vi "FestoCPX.File.Write.vi"(8 "error in":errorcluster, 11 "Settings dir":path) -> (0 "error out":errorcluster)   [LabVIEW 2016]
uses:
  FestoCPX.DO.Signal.ctl
  FestoCPX.DI.Signal.ctl
  FestoCPX.Global.vi
  <vilib>/Utility/config.llb/Write Key (I32).vi
  <vilib>/Utility/config.llb/Write Key (String).vi
  <vilib>/Utility/config.llb/NI_LVConfig.lvlib
panel:
  in  "DI Signal":T1
  in  "DO Signal":T2
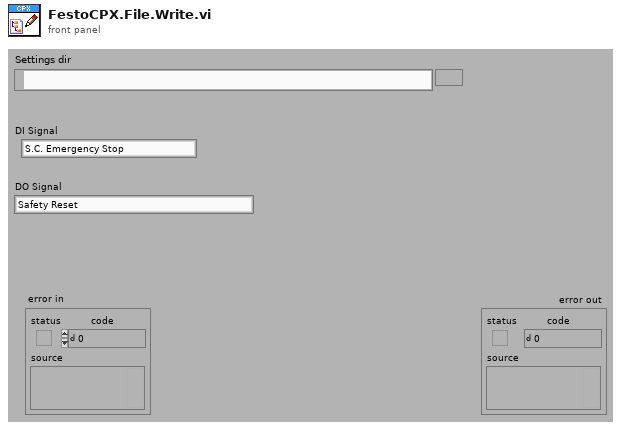
[diagram p1: front panel]
types:
  T1 = typedef "FestoCPX.DI.Signal.ctl" = enum16{"S.C. Emergency Stop", "S.C. Side Door Close", "S.C. Front Door Close", "S.C. Front Door Secured", "Button Start", "Button Stop", "Button Control", "Product Move Home", "Product Move Work", "Table Position", "Table Lock", "Product Lift A Home", "Product Lift B Home", "Product Arm OK", "Product Arm NOK", "Product Arm Work", "Revolver ID 1", "Revolver ID 2", "Revolver ID 3", "Revolver ID 4", "Revolver ID 5", "Air Pressure Inside", "Air Pressure Inlet", "Product Slot 1 A Present", "Product Slot 1 B Present", "Product Slot 2 A Present", "Product Slot 2 B Present", "Product Slot 3 A Present", "Product Slot 3 B Present", "Product Slot 4 A Present", "Product Slot 4 B Present", "Product Final A Present", "Product Final B Present", "Product Output A Present", "Product Output B Present", "Product Container OK Present", "Product Container NOK Present", "Fork ID 1", "Fork ID 2"}
  T2 = typedef "FestoCPX.DO.Signal.ctl" = enum16{"Safety Reset", "Air Main Valve", "Door Lock", "Button LED Start", "Button LED Stop", "Button LED Control", "Traffic LED Red", "Traffic LED Orange", "Traffic LED Green", "Horn", "Laser Interlock", "Laser Trigger", "Laser Fume Extractor", "Product Suction Gripper Slot 1 A", "Product Suction Gripper Slot 1 B", "Product Suction Gripper Slot 2 A", "Product Suction Gripper Slot 2 B", "Product Suction Gripper Slot 3 A", "Product Suction Gripper Slot 3 B", "Product Suction Gripper Slot 4 A", "Product Suction Gripper Slot 4 B", "Product Suction Gripper Final A", "Product Suction Gripper Final B", "Lamp", "Q1 Product Move Work", "Q1 Product Move Home", "Q2 Table Turn Work", "Q2 Table Turn Home", "Q3 Product Lift A", "Q3 Product Lift B", "Q4 Product Arm OK", "Q4 Product Arm NOK", "Q5 Product Arm Work", "Q6 Product BlowOut A", "Q6 Product BlowOut B"}
  T3 = typedef "FestoCPX.Data.Sets.ctl" = cluster{"IP":string, "Timeout_ms":i32, "ReconnectPeriod_s":i32, "Config.DI":T4[], "Config.DO":T6[]}
  T4 = typedef "FestoCPX.DI.Sets.ctl" = cluster{"Name":string, "Channel":T5, "Negate":bool}
  T5 = typedef "FestoCPX.DI.ctl" = enum16{"0.0", "0.1", "0.2", "0.3", "0.4", "0.5", "0.6", "0.7", "1.0", "1.1", "1.2", "1.3", "1.4", "1.5", "1.6", "1.7", "2.0", "2.1", "2.2", "2.3", "2.4", "2.5", "2.6", "2.7", "3.0", "3.1", "3.2", "3.3", "3.4", "3.5", "3.6", "3.7", "4.0", "4.1", "4.2", "4.3", "4.4", "4.5", "4.6", "4.7"}
  T6 = typedef "FestoCPX.DO.Sets.ctl" = cluster{"Name":string, "Channel":T7, "Negate":bool, "Default":bool}
  T7 = typedef "FestoCPX.DO.ctl" = enum16{"4.0", "4.1", "4.2", "4.3", "4.4", "4.5", "4.6", "4.7", "5.0", "5.1", "5.2", "5.3", "5.4", "5.5", "5.6", "5.7", "6.0", "6.1", "6.2", "6.3", "6.4", "6.5", "6.6", "6.7", "Q1K1", "Q1K2", "Q2K1", "Q2K2", "Q3K1", "Q3K2", "Q4K1", "Q4K2", "Q5K1", "Q5K2", "Q6K1", "Q6K2"}
  T8 = typedef "NI_LVConfig.lvlib/Config Data RefNum.ctl" = refnum<k1>
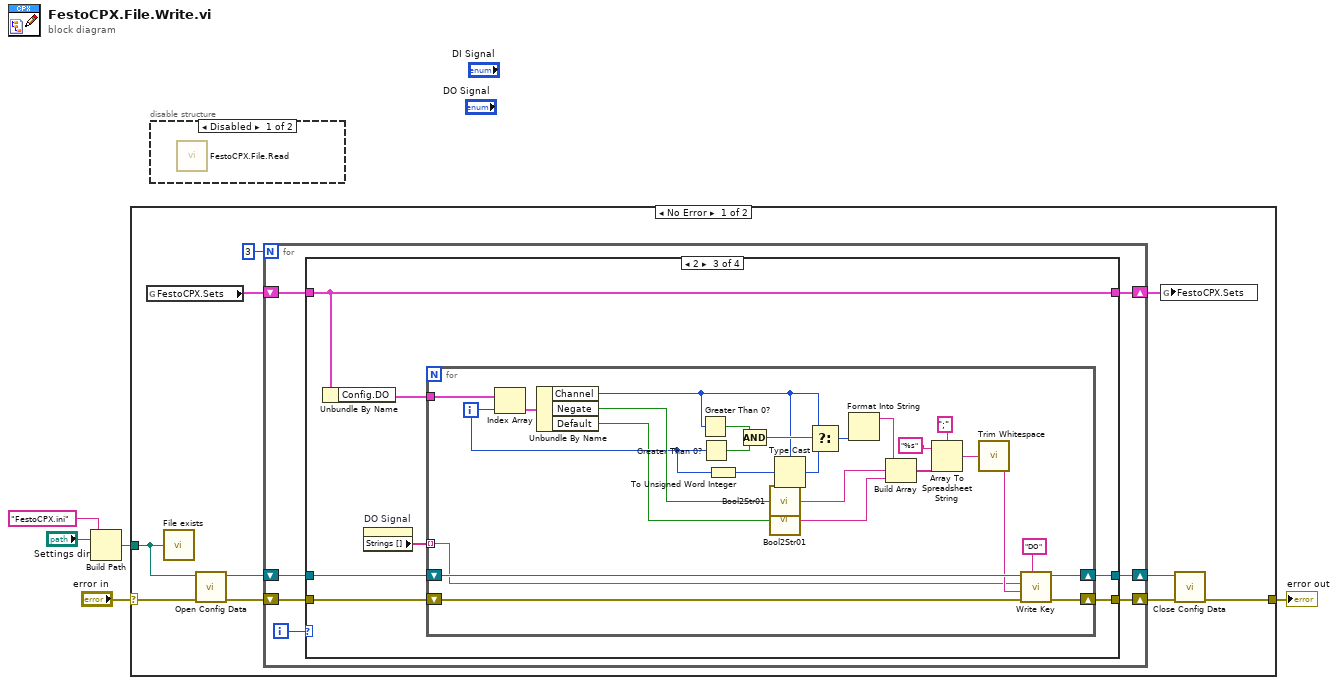
[diagram p0: block diagram]
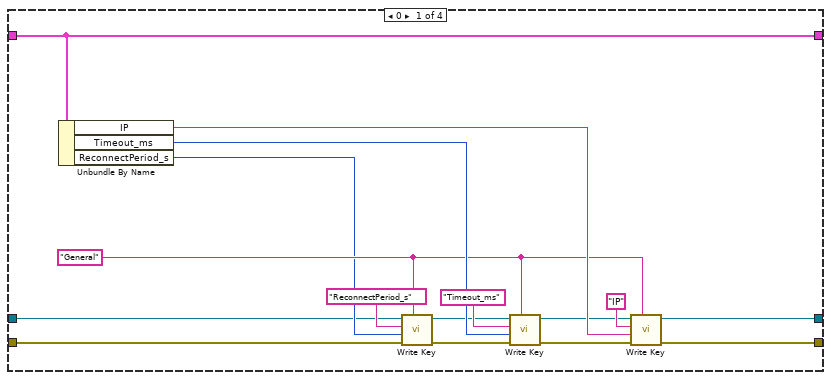
[diagram p3: hidden frame]
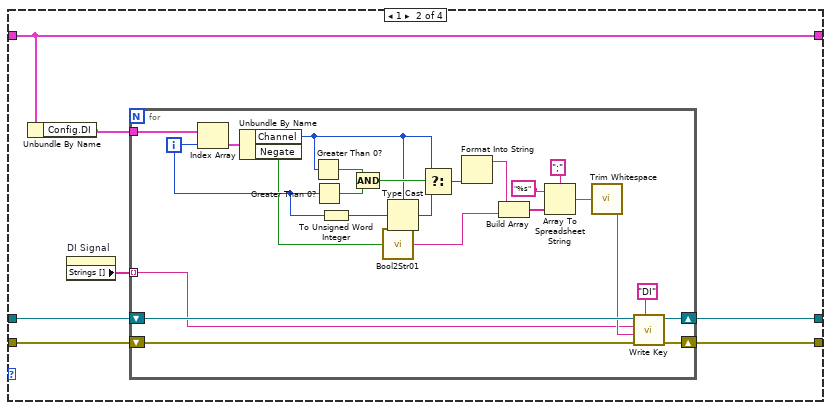
[diagram p4: hidden frame]
diagram:
  n1 = Build Path(base path="Settings dir", name or relative path="FestoCPX.ini") -> (appended path=w1:path)
  n2 = case shown="No Error" "error in" {
    selector: "error in" -> [w15 w106]
    tunnel: [w6 w106] -> w5
    tunnel: w1 -> [w14 _]
    frame No Error {
      n3 = global read "FestoCPX.Global.vi" "FestoCPX.Sets"() -> (w10:T3)
      n4 = call "File exists.vi"("file path"=w14) -> ()  [unwired: 4 in, 1 out]
      n5 = call <vilib>:"Open Config Data.vi"("error in (no error)"=w15, "configuration file path"=w14) -> ("error out"=w13:errorcluster, "refnum"=w12:T8)  [unwired: 7 in, 1 out]
      n6 = for {
        N: 3 -> [_]
        shift-right: [w19] -> w7
        shift-left: w12 -> [w21]
        shift-right: [w18] -> w8
        shift-left: w13 -> [w22]
        shift-right: [w17] -> w9
        shift-left: w10 -> [w16]
        i -> [w20]
        n7 = case shown="2" w20 {
          tunnel: w22 -> [w25 w45 w76 w105]
          tunnel: w21 -> [w24 w43 w74 w104]
          tunnel: [w33 w42 w73 w104] -> w19
          tunnel: [w32 w41 w72 w105] -> w18
          tunnel: [w37 w39 w70 w103] -> w17
          tunnel: w16 -> [w37 w39 w70 w103]
          frame 0 {
            w27 = "General" ("section")
            n8 = Unbundle By Name(w37) -> ("IP"=w35:string, "Timeout_ms"=w38:i32, "ReconnectPeriod_s"=w26:i32)
            n9 = call-poly <vilib>:"Write Key.vi"("section"=w27, "error in (no error)"=w25, "value"=w26, "key"="ReconnectPeriod_s", "refnum"=w24) -> ("error out"=w28:errorcluster, "refnum out"=w23:T8)  [unwired: 4 in, 1 out]
            n10 = call-poly <vilib>:"Write Key.vi"("section"=w27, "error in (no error)"=w28, "value"=w38, "key"="Timeout_ms", "refnum"=w23) -> ("error out"=w31:errorcluster, "refnum out"=w34:T8)  [unwired: 4 in, 1 out]
            n11 = call-poly <vilib>:"Write Key.vi"("section"=w27, "error in (no error)"=w31, "value"=w35, "key"="IP", "refnum"=w34) -> ("error out"=w32:errorcluster, "refnum out"=w33:T8)  [unwired: 4 in, 1 out]
          }
          frame 1 {
            n12 = Unbundle By Name(w39) -> ("Config.DI"=w40:T4[])
            n13 = property on="DI Signal" class="Enum (strict)"() -> ("Strings []"=w44:string[])  [unwired: 2 in, 2 out]
            n14 = for {
              tunnel: w44 -> [w46] mode=indexing
              tunnel: w40 -> [w63]
              shift-right: [w64] -> w41
              shift-left: w45 -> [w66]
              shift-right: [w65] -> w42
              shift-left: w43 -> [w67]
              i -> [w57]
              n15 = Index Array(array=w63, index=w57) -> (element=w61:T4)
              n16 = Unbundle By Name(w61) -> ("Channel"=w51:T5, "Negate"=w52:bool)
              n17 = Greater Than 0?(x=w51) -> (x > 0?=w60:bool)
              n18 = Greater Than 0?(x=w57) -> (x > 0?=w59:bool)
              n19 = To Unsigned Word Integer(number=w57) -> (unsigned 16bit integer=w56:u16)
              n20 = Compound Arithmetic op=AND(w60, w59) -> (w58:bool)
              n21 = call "Bool2Str01.vi"("Boolean"=w52) -> ("string"=w47:string)
              n22 = Type Cast(type=w51, x=w56) -> (*(type *) &x=w55:T5)
              n23 = Select(t=w51, s=w58, f=w55) -> (s? t:f=w54:T5)
              n24 = Format Into String(w54) -> (resulting string=w53:string)  [unwired: 3 in, 1 out]
              n25 = Build Array(w53, w47) -> (w50:string[])
              n26 = Array To Spreadsheet String(delimiter (Tab)=";", array=w50, 3:"%s" ("format string")) -> (spreadsheet string=w49:string)
              n27 = call <vilib>:"Trim Whitespace.vi"("string"=w49) -> ("trimmed string"=w48:string)  [unwired: 1 in]
              n28 = call-poly <vilib>:"Write Key.vi"("section"="DI", "error in (no error)"=w66, "value"=w48, "key"=w46, "refnum"=w67) -> ("error out"=w64:errorcluster, "refnum out"=w65:T8)  [unwired: 4 in, 1 out]
            }
          }
          frame 2 {
            n29 = Unbundle By Name(w70) -> ("Config.DO"=w71:T6[])
            n30 = property on="DO Signal" class="Enum (strict)"() -> ("Strings []"=w75:string[])  [unwired: 2 in, 2 out]
            n31 = for {
              tunnel: w75 -> [w82] mode=indexing
              tunnel: w71 -> [w96]
              shift-right: [w97] -> w72
              shift-left: w76 -> [w99]
              shift-right: [w98] -> w73
              shift-left: w74 -> [w100]
              i -> [w79]
              n32 = Index Array(array=w96, index=w79) -> (element=w94:T6)
              n33 = Unbundle By Name(w94) -> ("Channel"=w86:T7, "Negate"=w81:bool, "Default"=w78:bool)
              n34 = Greater Than 0?(x=w86) -> (x > 0?=w93:bool)
              n35 = Greater Than 0?(x=w79) -> (x > 0?=w92:bool)
              n36 = To Unsigned Word Integer(number=w79) -> (unsigned 16bit integer=w90:u16)
              n37 = Compound Arithmetic op=AND(w93, w92) -> (w91:bool)
              n38 = call "Bool2Str01.vi"("Boolean"=w81) -> ("string"=w80:string)
              n39 = call "Bool2Str01.vi"("Boolean"=w78) -> ("string"=w77:string)
              n40 = Type Cast(type=w86, x=w90) -> (*(type *) &x=w89:T7)
              n41 = Select(t=w86, s=w91, f=w89) -> (s? t:f=w88:T7)
              n42 = Format Into String(w88) -> (resulting string=w87:string)  [unwired: 3 in, 1 out]
              n43 = Build Array(w87, w80, w77) -> (w85:string[])
              n44 = Array To Spreadsheet String(delimiter (Tab)=";", array=w85, 3:"%s" ("format string")) -> (spreadsheet string=w84:string)
              n45 = call <vilib>:"Trim Whitespace.vi"("string"=w84) -> ("trimmed string"=w83:string)  [unwired: 1 in]
              n46 = call-poly <vilib>:"Write Key.vi"("section"="DO", "error in (no error)"=w99, "value"=w83, "key"=w82, "refnum"=w100) -> ("error out"=w97:errorcluster, "refnum out"=w98:T8)  [unwired: 4 in, 1 out]
            }
          }
          frame Default {
          }
        }
      }
      n47 = global write "FestoCPX.Global.vi" "FestoCPX.Sets"(w9) -> ()
      n48 = call <vilib>:"Close Config Data.vi"("error in (no error)"=w8, "refnum"=w7) -> ("error out"=w6:errorcluster)  [unwired: 8 in, 1 out]
    }
    frame Error {
    }
  }
  "error out" <- w5
  n49 = disable-structure shown="Disabled" {
    frame Disabled {
      n50 = call "FestoCPX.File.Read.vi"() -> ()  [unwired: 11 in, 1 out]
    }
    frame Enabled {
    }
  }
